vi "CMD.vi"(0 "class data in":refnum<class "MB_ENGINE.lvclass">, 5 "cmd to write":T1 items=["0 Idle"=0, "1 GoTo Absolute Position"=1, "2 GoTo Relative"=2, "10 GoTo Home Position"=10, "11 Set Home Position"=11, "12 Set FindHome Mode"=12, "13 Reset FindHome Mode"=13, "14 Get FindHome State"=14, "20 Hard Stop"=20, "21 HiZ Stop"=21, "22 Soft Stop"=22, "30 Clear Fault"=30, "40 Encoder Set Home"=40, "70 Driver Init"=70], 11 "error in (no error)":errorcluster) -> (4 "class data out":refnum<class "MB_ENGINE.lvclass">, 15 "error out":errorcluster)   [LabVIEW 2019, in "MB_ENGINE.lvclass"]
uses:
  MB_ENGINE.lvclass
  cmd enum.ctl
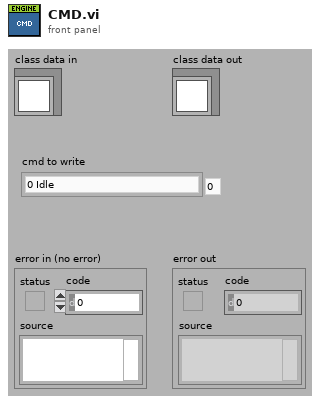
[diagram p1: front panel]
types:
  T1 = typedef "MB_ENGINE.lvclass/cmd enum.ctl" = u16
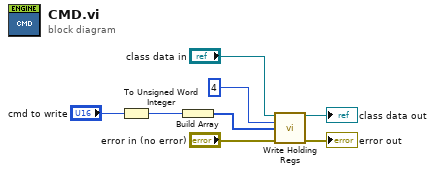
[diagram p0: block diagram]
diagram:
  n1 = To Unsigned Word Integer(number="cmd to write") -> (unsigned 16bit integer=w3:T1)
  n2 = Build Array(w3) -> (w2:T1[])
  n3 = call-dynamic "Write Holding Regs.vi"("reference in"="class data in", "starting address"=u16 4, "Regs"=w2, "error in (no error)"="error in (no error)") -> ("reference out"=→"class data out":refnum<class "MB_ENGINE.lvclass">, "error out"=→"error out":errorcluster)  [unwired: 10 in]
